vi "Enqueue - ClusterBoth.vi"(5 "Insert? (T)":bool=TRUE, 7 "At Front? (F)":bool, 8 "error in (no error)":errorcluster, 9 "Data":variant, 10 "Command":string, 11 "Queue with Cluster Reference":T1) -> (0 "error out":errorcluster, 3 "Queue Out (dup)":T1)   [LabVIEW 2010]
doc: "This VI enqueues a command and data cluster into the referenced queue.\n\nInputs:\nQueue with Cluster Reference - (queue) queue to insert cluster into\nCommand - (string) command part of the cluster to be inserted into the queue (may have arguments)\nData - (var) data part of the cluster to be inserted into the queue\nAt Front? (F) - (bool) set TRUE to insert cluster at the beginning of the queue; FALSE (default) at the end\nInsert? (T) - (bool) TRUE = insert cluster into queue (default); FALSE = do not insert cluster (controlled via logic)\nerror in - error input cluster\n\nOutputs:\nQueue Out (dup) - (queue) duplicate reference to input queue\nerror out - error output cluster"
uses:
  <userlib>/Common/Queue with Cluster/TYP_Queue with Cluster Reference.ctl
panel:
  # "Inputs"
  # "Outputs"
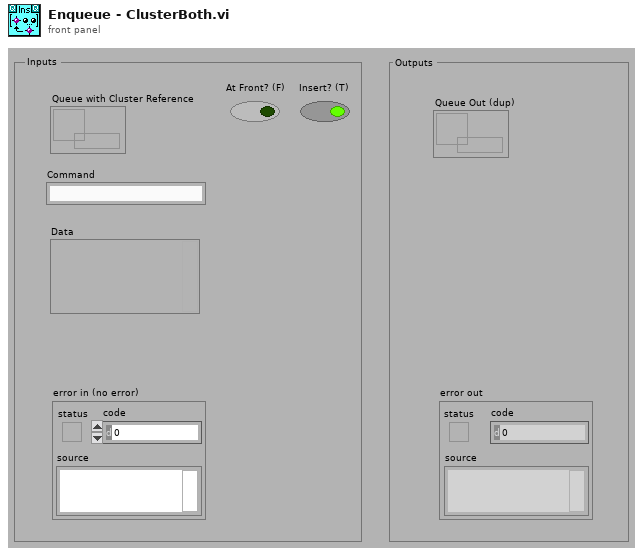
[diagram p1: front panel]
types:
  T1 = typedef "TYP_Queue with Cluster Reference.ctl" = refnum<queue>
  T2 = typedef "TYP_Queue Cluster Element.ctl" = cluster{"Command":string, "Data":variant}
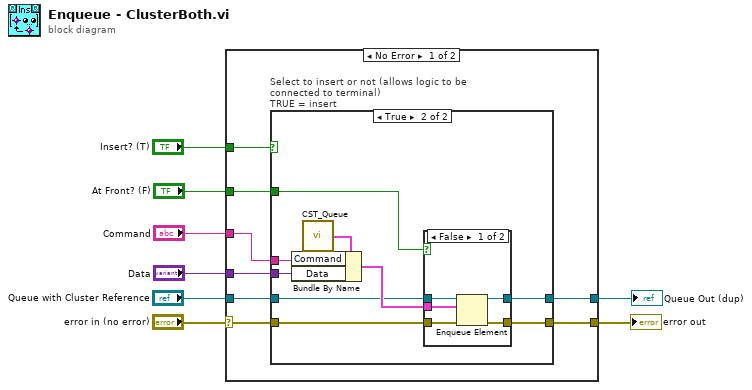
[diagram p0: block diagram]
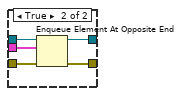
[diagram p3: hidden frame]
diagram:
  n1 = case shown="No Error" "error in (no error)" {
    selector: "error in (no error)" -> [w11 w39]
    tunnel: [w15 w39] -> w7
    tunnel: "Command" -> [w12 _]
    tunnel: "Data" -> [w14 _]
    tunnel: "Queue with Cluster Reference" -> [w16 w38]
    tunnel: [w13 w38] -> w3
    tunnel: "At Front? (F)" -> [w10 _]
    tunnel: "Insert? (T)" -> [w9 _]
    frame No Error {
      n2 = case "Select to insert or not (allows logic to be connected to terminal)\nTRUE = insert" shown="True" w9 {
        tunnel: w16 -> [w18 w25]
        tunnel: [w17 w24] -> w15
        tunnel: w14 -> [_ w23]
        tunnel: [w18 w22] -> w13
        tunnel: w12 -> [_ w21]
        tunnel: w11 -> [w17 w20]
        tunnel: w10 -> [_ w19]
        frame False {
        }
        frame True {
          n3 = call <userlib>:"CST_Queue.vi"() -> ("Queue Cluster Element"=w27:T2)  [unwired: 1 in]
          n4 = Bundle By Name(cluster=w27, "Command"=w21, "Data"=w23) -> (w26:T2)
          n5 = case shown="False" w19 {
            tunnel: w26 -> [w32 w36]
            tunnel: w25 -> [w31 w37]
            tunnel: [w30 w33] -> w24
            tunnel: [w29 w34] -> w22
            tunnel: w20 -> [w28 w35]
            frame False {
              n6 = Enqueue Element(queue=w31, element=w32, error in (no error)=w28) -> (queue out=w29:T1, error out=w30:errorcluster)  [unwired: 1 in, 1 out]
            }
            frame True {
              n7 = Enqueue Element At Opposite End(queue=w37, element=w36, error in (no error)=w35) -> (queue out=w34:T1, error out=w33:errorcluster)  [unwired: 1 in, 1 out]
            }
          }
        }
      }
    }
    frame Error {
    }
  }
  "error out" <- w7
  "Queue Out (dup)" <- w3
